vi "Get Component Collision.vi"(11 "Collision in":refnum<class "Collision.lvclass">) -> (1 "Movable out":refnum<class "Movable.lvclass">, 2 "GB Component out":refnum<class "Game Board Component.lvclass">)   [LabVIEW 2021, in "Collision.lvclass"]
doc: "MIT Licence\nCopyright (c) 2024 David Grollier"
uses:
  Collision.lvclass
  Game Componants/Game Board Component/Movable/Movable.lvclass
  Game Componants/Game Board Component/Game Board Component.lvclass
  Collision.lvclass/Collision.ctl
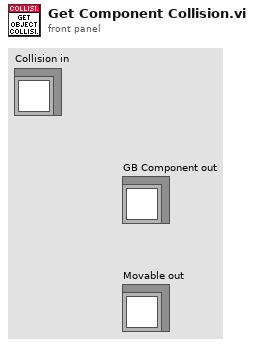
[diagram p1: front panel]
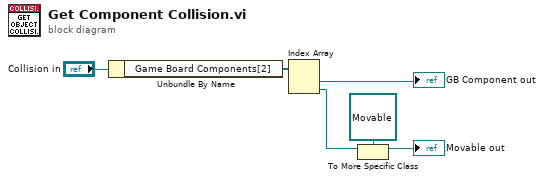
[diagram p0: block diagram]
diagram:
  n1 = Unbundle By Name("Collision in") -> ("Game Board Components[2]"=w5:refnum<class "Game Board Component.lvclass">[])
  n2 = Index Array(array=w5) -> (element #1=→"GB Component out":refnum<class "Game Board Component.lvclass">, element #2=w3:refnum<class "Game Board Component.lvclass">)  [unwired: 2 in]
  n3 = To More Specific Class(target class=refnum<class "Movable.lvclass"> refnum ("Movable.lvclass"), reference=w3) -> (specific class reference=→"Movable out":refnum<class "Movable.lvclass">)  [unwired: 1 in, 1 out]
